vi "WaterfallSelect.vi"(8 "error in":errorcluster, 11 "WaterfallSelect(0-4)":u8) -> (0 "error out":errorcluster)   [LabVIEW 2018, in "Vibration.lvlib"]
doc: "This subVI enqueues the named action in to the communications queue along with the input data."
uses:
  Vibration.lvlib
  Private Controls/Module Data.ctl
  Private Controls/Module Action.ctl
  fee29557-b1a7-4563-b595-d77072d98f74.vi
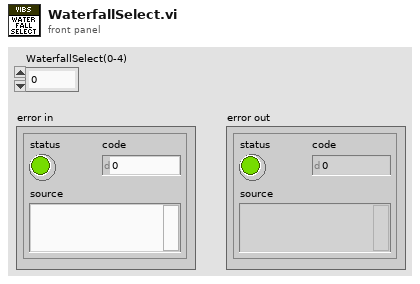
[diagram p1: front panel]
types:
  T1 = typedef "Vibration.lvlib/Module Data.ctl" = cluster{"Data":variant, "Action":T2}
  T2 = typedef "Vibration.lvlib/Module Action.ctl" = enum16{"Init", "Waterfall Select", "Read", "Accel Sensitivities", "Filters", "Error"}
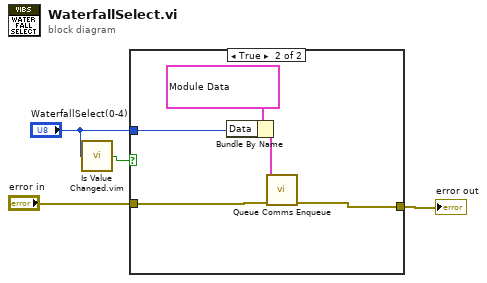
[diagram p0: block diagram]
diagram:
  n1 = call "Is Value Changed.vim"("value"="WaterfallSelect(0-4)") -> ("changed or first call?"=w2:bool)
  n2 = case shown="True" w2 {
    tunnel: [w5 w10] -> w4
    tunnel: "error in" -> [w5 w9]
    tunnel: "WaterfallSelect(0-4)" -> [_ w6]
    frame False {
    }
    frame True {
      n3 = Bundle By Name(cluster=T1 {"Data"=variant, "Action"=enum."Waterfall Select"} ("element"), "Data"=w6) -> (w7:T1)
      n4 = call "Queue Comms Enqueue.vi"("error in (no error)"=w9, "element"=w7) -> ("error out"=w10:errorcluster)  [unwired: 9 in]
    }
  }
  "error out" <- w4
